vi "Get Supported Targets.vi"(8 "error in":errorcluster, 11 "configuration in":refnum<class "PL_Target Configuration.lvclass">) -> (0 "error out":errorcluster, 2 "supported targets":T1[](array[typedef]), 3 "configuration out":refnum<class "PL_Target Configuration.lvclass">)   [LabVIEW 2013, in "PL_Target Configuration.lvclass"]
doc: "Provides an interface for determining the targets supported by a given configuration/runtime class pairing. This should be overridden by any useful child class."
uses:
  PL_Target Configuration.lvclass
  <vilib>/NI/Tag Bus Module Framework/root configuration/Target Types.ctl
  <vilib>/NI/Tag Bus Module Framework/root configuration/TBM configuration.lvclass
  <vilib>/NI/CEF/CEF_TreeControl/serializable configuration/NISE_CEF_serializable configuration.lvclass
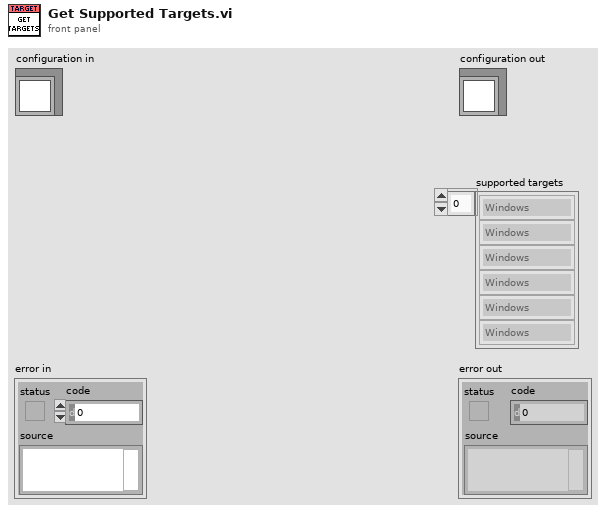
[diagram p1: front panel]
types:
  T1 = typedef "TBM configuration.lvclass/Target Types.ctl" = enum16{"Windows", "Mac", "Linux", "Linux RT ARM", "VxWorks", "Pharlap", "Other", "Linux RT x64"}
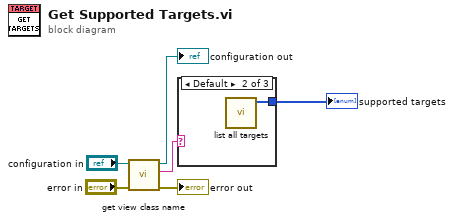
[diagram p0: block diagram]
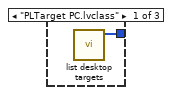
[diagram p2: hidden frame]
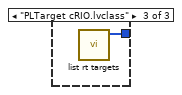
[diagram p3: hidden frame]
diagram:
  n1 = call <vilib>:"get view class name.vi"("error in"="error in", "configuration in"="configuration in") -> ("error out"=→"error out":errorcluster, "view class"=w5:string, "configuration out"=→"configuration out":refnum<class "PL_Target Configuration.lvclass">)  [unwired: 7 in]
  n2 = case shown="Default" w5 {
    tunnel: [w7 w8 w9] -> w6
    frame "PLTarget PC.lvclass" {
      n3 = call <vilib>:"list desktop targets.vi"() -> ("desktop targets"=w7:T1[])  [unwired: 11 in]
    }
    frame Default {
      n4 = call <vilib>:"list all targets.vi"() -> ("all targets"=w8:T1[])  [unwired: 11 in]
    }
    frame "PLTarget cRIO.lvclass" {
      n5 = call <vilib>:"list rt targets.vi"() -> ("desktop targets"=w9:T1[])  [unwired: 11 in]
    }
  }
  "supported targets" <- w6
